vi "Read Bus Monitor Log.vi"(5 "Component ID":u8, 7 "FPGA Interface":refnum<class "FPGA Interface.lvclass">, 8 "error in (no error)":errorcluster, 11 "Bus Monitor in":refnum<class "Bus Monitor.lvclass">) -> (0 "error out":errorcluster, 1 "Bus B Monitor Log":string[][](array[string]), 2 "Bus A Monitor Log":string[][](array[string]), 3 "Bus Monitor out":refnum<class "Bus Monitor.lvclass">)   [LabVIEW 2016, in "BCI-1553 API.lvlib" / "Bus Monitor.lvclass"]
doc: "Read the current log stored by the bus monitor for both Bus A and Bus B. Depending on the data rates in the system, these logs may roll-over at various times in the application execution."
uses:
  Bus Monitor.lvclass
  Dependencies/FPGA Interface/FPGA Interface.lvclass
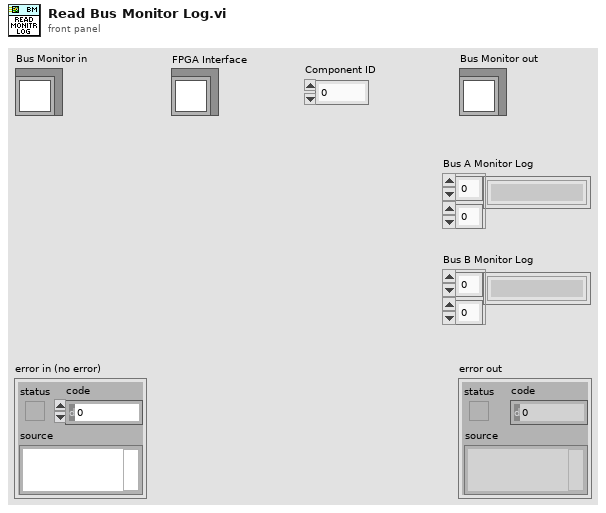
[diagram p1: front panel]
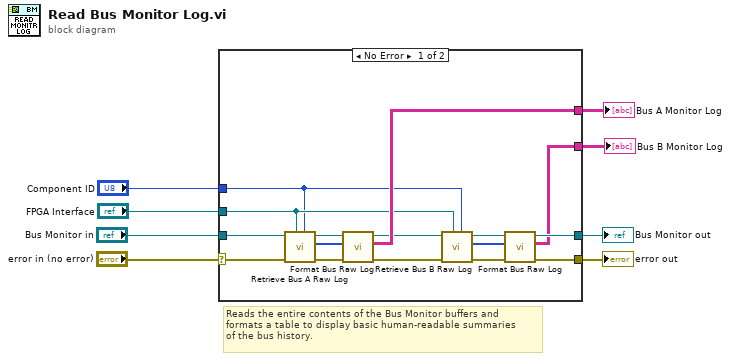
[diagram p0: block diagram]
diagram:
  # "Reads the entire contents of the Bus Monitor buffers and\nformats a table to display basic human-readable summaries\nof the bus history."
  n1 = case shown="No Error" "error in (no error)" {
    selector: "error in (no error)" -> [w23 w26]
    tunnel: [w13 w26] -> w7
    tunnel: [w14 w25] -> w5
    tunnel: "Bus Monitor in" -> [w24 w25]
    tunnel: "FPGA Interface" -> [w16 _]
    tunnel: "Component ID" -> [w15 _]
    tunnel: [w19 _] -> w2
    tunnel: [w12 _] -> w1
    frame No Error {
      n2 = call "Retrieve Bus A Raw Log.vi"("Component ID"=w15, "FPGA Interface"=w16, "error in (no error)"=w23, "Bus Monitor in"=w24) -> ("error out"=w22:errorcluster, "Bus A Raw Log"=w20:u16[], "Bus Monitor out"=w21:refnum<class "Bus Monitor.lvclass">)  [unwired: 5 in]
      n3 = call "Format Bus Raw Log.vi"("error in (no error)"=w22, "Bus Raw Log"=w20, "Bus Monitor in"=w21) -> ("error out"=w18:errorcluster, "Formatted Log"=w19:string[][], "Bus Monitor out"=w17:refnum<class "Bus Monitor.lvclass">)  [unwired: 6 in]
      n4 = call "Retrieve Bus B Raw Log.vi"("Component ID"=w15, "FPGA Interface"=w16, "error in (no error)"=w18, "Bus Monitor in"=w17) -> ("error out"=w10:errorcluster, "Bus A Raw Log"=w9:u16[], "Bus Monitor out"=w11:refnum<class "Bus Monitor.lvclass">)  [unwired: 5 in]
      n5 = call "Format Bus Raw Log.vi"("error in (no error)"=w10, "Bus Raw Log"=w9, "Bus Monitor in"=w11) -> ("error out"=w13:errorcluster, "Formatted Log"=w12:string[][], "Bus Monitor out"=w14:refnum<class "Bus Monitor.lvclass">)  [unwired: 6 in]
    }
    frame Error {
    }
  }
  "error out" <- w7
  "Bus Monitor out" <- w5
  "Bus A Monitor Log" <- w2
  "Bus B Monitor Log" <- w1
